vi "New Results (to override).vi"(8 "error in (no error)":errorcluster, 9 "Results In":refnum<class "Analyze Results Base.lvclass">[](array[class]), 10 "Parameters":refnum<class "Analyze Parameter Base.lvclass">[](array[class]), 11 "Launch IMAQ Display in":refnum<class "HIJ Vision File Viewer App.lvclass">) -> (0 "error out":errorcluster, 3 "Launch IMAQ Display out":refnum<class "HIJ Vision File Viewer App.lvclass">)   [LabVIEW 2014, in "HIJ Vision File Viewer App.lvlib" / "HIJ Vision File Viewer App.lvclass"]
uses:
  HIJ Vision File Viewer App.lvclass
  Analyze/Results and Overlays/Results Base/Analyze Results Base.lvclass
  Analyze/Analyze Parameter/Analyze Parameter Base/Analyze Parameter Base.lvclass
  HIJ Vision File Viewer App.lvclass/HIJ Vision File Viewer App.ctl
  HIJ Vision Application/HIJ Vision Application/HIJ Vision Application.lvclass
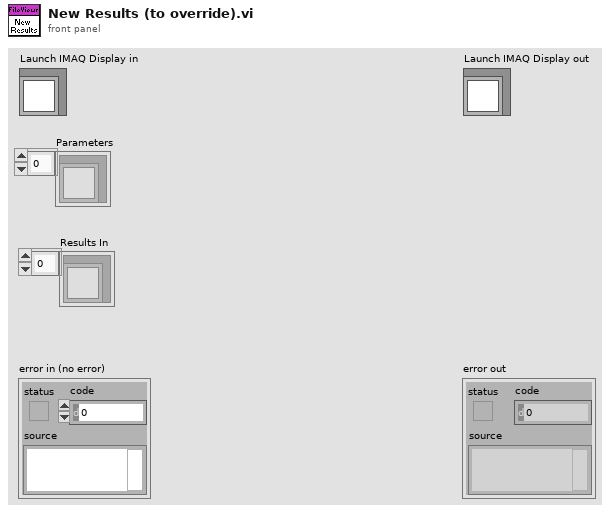
[diagram p1: front panel]
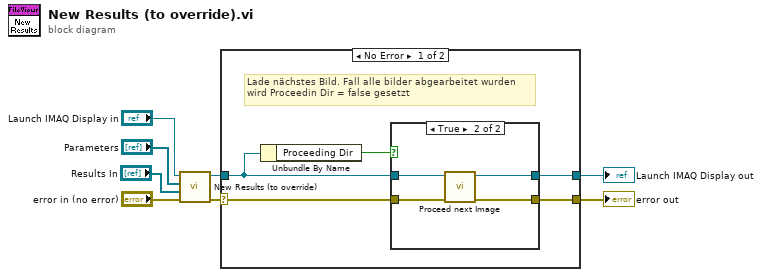
[diagram p0: block diagram]
diagram:
  n1 = call-parent "New Results (to override).vi"("error in (no error)"="error in (no error)", "Results In"="Results In", "Parameters"="Parameters", "Launch IMAQ Display in"="Launch IMAQ Display in") -> ("error out"=w1:errorcluster, "Launch IMAQ Display out"=w3:refnum<class "HIJ Vision File Viewer App.lvclass">)  [unwired: 6 in]
  n2 = case shown="No Error" w1 {
    selector: w1 -> [w9 w21]
    tunnel: [w13 w20] -> w4
    tunnel: w3 -> [w12 w20]
    tunnel: [w11 w21] -> w2
    frame No Error {
      # "Lade nächstes Bild. Fall alle bilder abgearbeitet wurden\nwird Proceedin Dir = false gesetzt"
      n3 = Unbundle By Name(w12) -> ("Proceeding Dir"=w10:bool)
      n4 = case shown="True" w10 {
        tunnel: [w15 w19] -> w13
        tunnel: w12 -> [w15 w18]
        tunnel: w9 -> [w14 w17]
        tunnel: [w14 w16] -> w11
        frame False {
        }
        frame True {
          n5 = call-dynamic "Proceed next Image.vi"("error in (no error)"=w17, "Launch File Viewer in"=w18) -> ("error out"=w16:errorcluster, "Launch File Viewer out"=w19:refnum<class "HIJ Vision File Viewer App.lvclass">)  [unwired: 8 in]
        }
      }
    }
    frame Error {
    }
  }
  "error out" <- w2
  "Launch IMAQ Display out" <- w4
